vi "jv_keithley-2450_python.vi"(5 "Cell details cluster":T1={"Cell Position"=16, "Cell Label"="", "Pixel to measure"=0, "Area (cm^2)"=0.126, "Variable"="", "Variable value"="", "Scan settings in queue"=0, "Light or dark"="", "Measurement type"=""} {"Pixel to measure" items=["All", "1", "2", "3", "4", "5", "6", "7", "8"]}, 6 "intensity (# of suns)":string, 7 "Scan settings":T2={"J-V scan"=TRUE, "Start voltage (V)"=0.0, "End voltage (V)"=0.0, "Step voltage (V)"=1.4, "Scan both directions"=TRUE, "Inverted device structure"=FALSE, "Measurement delay (ms)"=10.0, "Measurement speed"=0, "Scan rate (V/s)"=0.0, "Stabilisation time (s)"=0.0, "Stabilisation mode"=0, "Stabilisation value (V or A) "=1.0, "Illumination"=0, "Stabilisation in the dark?"=FALSE, "Repeat light scans"=FALSE, "No. of repeat scans"=0.0, "Only repeat for best pixel"=1, "J-t scan"=FALSE, "J-t best pixel only"=7, "J-t start voltage (V)"=0.0, "J-t end voltage (V)"=1.4, "J-t step voltage (V)"=0.01, "Step time (s)"=0.7, "J-t scan both directions"=TRUE, "J-t inverted device structure"=FALSE, "Settling delay (s)"=0.0, "J-t measurement speed"=0, "J-t illumination"=2, "Max. power stabilisation"=FALSE, "Max power best pixel only"=1, "Max. power point tracker"=FALSE, "Vmp from J-V scan"=FALSE, "Max P stab. Specific voltage"=FALSE, "Vmp (V)"=1.0, "Stabilisation time step (s)"=1.0, "Total stabilisation time (s)"=100.0} {"Settling delay (s)" min=0.0; "J-t illumination" items=["Light only", "Dark only", "Light then dark", "Dark then light"]; "Measurement speed" items=["Fast", "Normal", "High accuracy"]; "Illumination" items=["Light only", "Dark only", "Light then dark", "Dark then light"]; "Only repeat for best pixel" items=["only for best pixel", "for best 2 pixels", "for best 3 pixels", "for best 4 pixels", "for best 5 pixels", "for best 6 pixels", "for best 7 pixels", "for all pixels"]; "No. of repeat scans" min=1.0 step=1.0; "Max power best pixel only" items=["only the best pixel", "the best 2 pixels", "the best 3 pixels", "the best 4 pixels", "the best 5 pixels", "the best 6 pixels", "the best 7 pixels", "all pixels"]; "J-t best pixel only" items=["only the best pixel", "the best 2 pixels", "the best 3 pixels", "the best 4 pixels", "the best 5 pixels", "the best 6 pixels", "the best 7 pixels", "all pixels"]; "J-t measurement speed" items=["Fast", "Normal", "High Accuracy"]; "Stabilisation mode" items=["V", "I"]; "Measurement delay (ms)" min=10.0}, 8 "error in (no error)":errorcluster, 10 "file name":string, 11 "folder path":string) -> (0 "error out":errorcluster, 1 "1st scan direction":string, 2 "HL j-v metrics":string[](array[string]), 3 "LH j-v metrics":string[](array[string]))   [LabVIEW 2016]
uses:
  TypeDefs/scan_settings.ctl
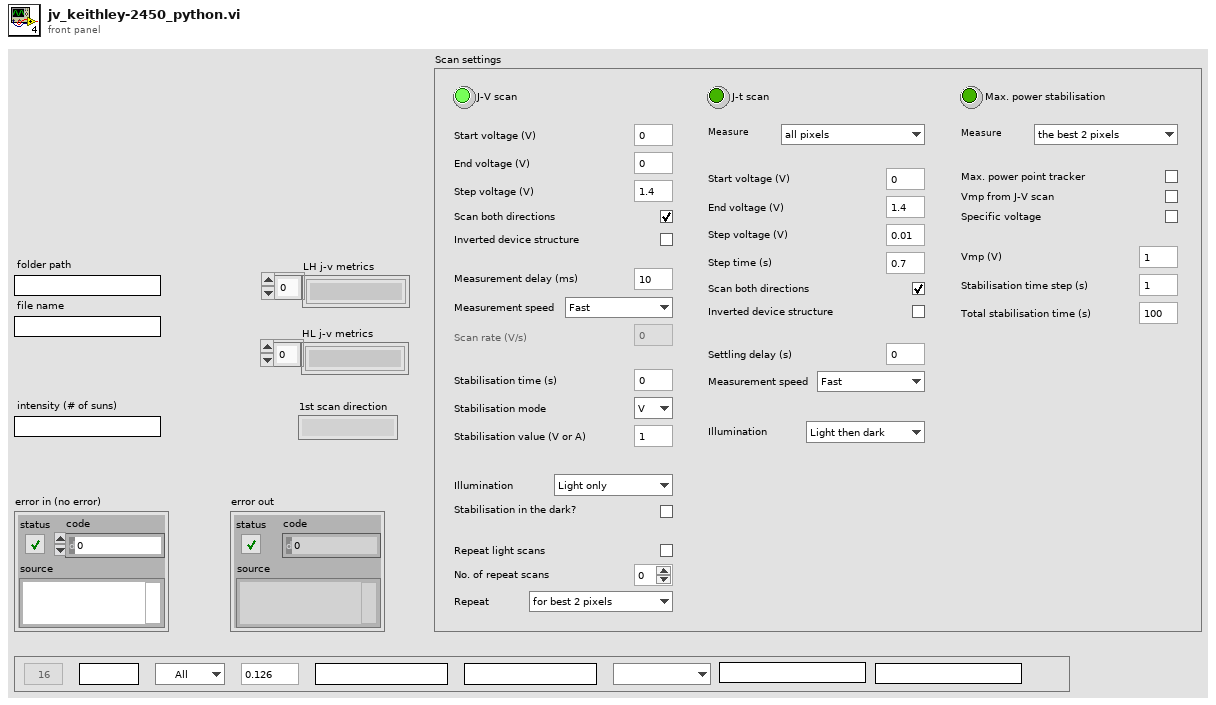
[diagram p1: front panel]
types:
  T1 = cluster{"Cell Position":i32, "Cell Label":string, "Pixel to measure":u16, "Area (cm^2)":dbl, "Variable":string, "Variable value":string, "Scan settings in queue":u16, "Light or dark":string, "Measurement type":string}
  T2 = typedef "scan_settings.ctl" = cluster{"J-V scan":bool, "Start voltage (V)":dbl, "End voltage (V)":dbl, "Step voltage (V)":dbl, "Scan both directions":bool, "Inverted device structure":bool, "Measurement delay (ms)":dbl, "Measurement speed":u8, "Scan rate (V/s)":dbl, "Stabilisation time (s)":dbl, "Stabilisation mode":u16, "Stabilisation value (V or A) ":dbl, "Illumination":u16, "Stabilisation in the dark?":bool, "Repeat light scans":bool, "No. of repeat scans":dbl, "Only repeat for best pixel":u16, "J-t scan":bool, "J-t best pixel only":u16, "J-t start voltage (V)":dbl, "J-t end voltage (V)":dbl, "J-t step voltage (V)":dbl, "Step time (s)":dbl, "J-t scan both directions":bool, "J-t inverted device structure":bool, "Settling delay (s)":dbl, "J-t measurement speed":u16, "J-t illumination":u16, "Max. power stabilisation":bool, "Max power best pixel only":u16, "Max. power point tracker":bool, "Vmp from J-V scan":bool, "Max P stab. Specific voltage":bool, "Vmp (V)":dbl, "Stabilisation time step (s)":dbl, "Total stabilisation time (s)":dbl}
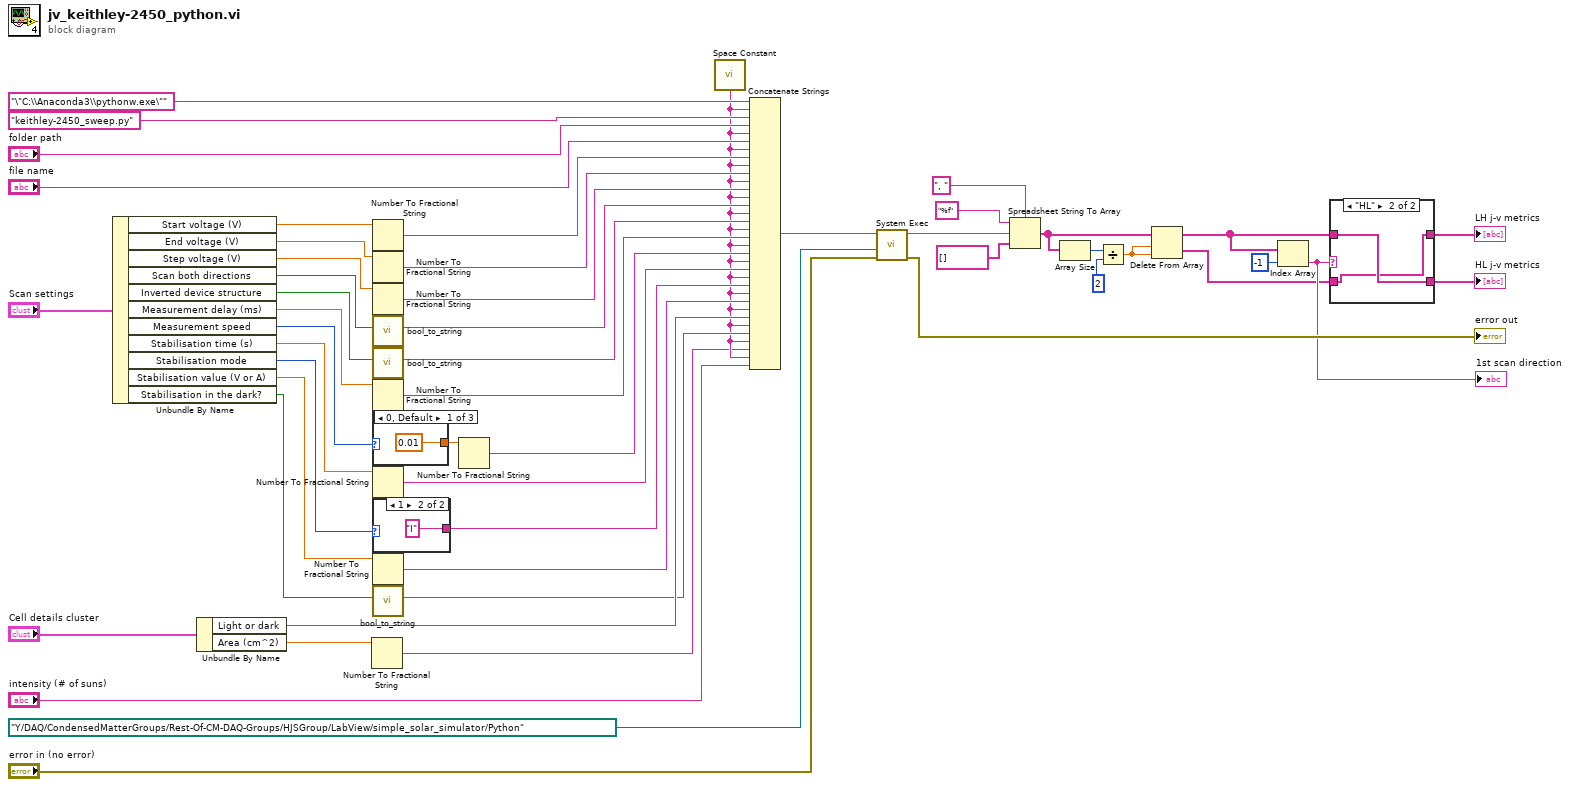
[diagram p0: block diagram]
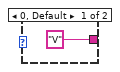
[diagram p3: hidden frame]
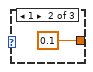
[diagram p4: hidden frame]
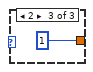
[diagram p5: hidden frame]
diagram:
  n1 = Unbundle By Name("Scan settings") -> ("Start voltage (V)"=w45:dbl, "End voltage (V)"=w44:dbl, "Step voltage (V)"=w43:dbl, "Scan both directions"=w42:bool, "Inverted device structure"=w41:bool, "Measurement delay (ms)"=w40:dbl, "Measurement speed"=w39:u8, "Stabilisation time (s)"=w37:dbl, "Stabilisation mode"=w36:u16, "Stabilisation value (V or A)"=w35:dbl, "Stabilisation in the dark?"=w34:bool)
  n2 = Unbundle By Name("Cell details cluster") -> ("Light or dark"=w23:string, "Area (cm^2)"=w8:dbl)
  n3 = Number To Fractional String(number=w8) -> (F-format string=w7:string)  [unwired: 3 in]
  n4 = Number To Fractional String(number=w45) -> (F-format string=w33:string)  [unwired: 3 in]
  n5 = Number To Fractional String(number=w44) -> (F-format string=w32:string)  [unwired: 3 in]
  n6 = Number To Fractional String(number=w43) -> (F-format string=w31:string)  [unwired: 3 in]
  n7 = call "bool_to_string.vi"("Boolean"=w42) -> ("String"=w30:string)  [unwired: 10 in]
  n8 = call "bool_to_string.vi"("Boolean"=w41) -> ("String"=w29:string)  [unwired: 10 in]
  n9 = Number To Fractional String(number=w40) -> (F-format string=w28:string)  [unwired: 3 in]
  n10 = case shown="0, Default" w39 {
    tunnel: [0.01 0.1 1] -> w38
    frame 0, Default {
    }
    frame 1 {
    }
    frame 2 {
    }
  }
  n11 = Number To Fractional String(number=w37) -> (F-format string=w26:string)  [unwired: 3 in]
  n12 = case shown="1" w36 {
    tunnel: ["V" "I"] -> w25
    frame 0, Default {
    }
    frame 1 {
    }
  }
  n13 = Number To Fractional String(number=w35) -> (F-format string=w24:string)  [unwired: 3 in]
  n14 = call "bool_to_string.vi"("Boolean"=w34) -> ("String"=w22:string)  [unwired: 10 in]
  n15 = Number To Fractional String(number=w38) -> (F-format string=w27:string)  [unwired: 3 in]
  n16 = call <vilib>:"Space Constant.vi"() -> ("String"=w21:string)
  n17 = Concatenate Strings("\"C:\\Anaconda3\\pythonw.exe\"" ("standard input"), w21, "keithley-2450_sweep.py" ("standard input"), "folder path", w21, "file name", w21, w33, w21, w32, w21, w31, w21, w30, w21, w29, w21, w28, w21, w27, w21, w26, w21, w25, w21, w24, w21, w23, w21, w22, w21, w7, w21, "intensity (# of suns)") -> (w50:string)
  n18 = call <vilib>:"System Exec.vi"("error in (no error)"="error in (no error)", "working directory"=path "Y:/DAQ/CondensedMatterGroups/Rest-Of-CM-DAQ-Groups/HJSGroup/LabView/simple_solar_simulator/Python", "command line"=w50) -> ("error out"=→"error out":errorcluster, "standard output"=w14:string)  [unwired: 5 in, 2 out]
  n19 = Spreadsheet String To Array(delimiter (Tab)=", ", format string="%f", spreadsheet string=w14, array type (2D Dbl)=string[] []) -> (array=w13:string[])
  n20 = Array Size(array=w13) -> (size(s)=w12:i32)
  n21 = Divide(x=w12, y=2) -> (x/y=w10:dbl)
  n22 = Delete From Array(array=w13, length=w10, index=w10) -> (deleted portion=w1:string[], array with subset deleted=w4:string[])
  n23 = Index Array(array=w4, index=-1) -> (element=w5:string)
  "1st scan direction" <- w5
  n24 = case shown="\"HL\"" w5 {
    tunnel: w4 -> [w59 w61]
    tunnel: [w59 w60] -> w3
    tunnel: [w58 w61] -> w2
    tunnel: w1 -> [w58 w60]
    frame "LH", Default {
    }
    frame "HL" {
    }
  }
  "LH j-v metrics" <- w3
  "HL j-v metrics" <- w2
